vi "Fetch (PV Data).vi"(7 "PV name":string, 8 "error in":errorcluster, 11 "Source in":refnum<class "Source.lvclass">) -> (0 "error out":errorcluster, 1 "PV found?":bool, 2 "PV Data out":refnum<class "PV Data.lvclass">, 3 "Source out":refnum<class "Source.lvclass">)   [LabVIEW 2020, in "PV Access.lvlib" / "PVA Server.lvlib" / "Source.lvclass"]
uses:
  Source.lvclass
  PV Data/PV Data/PV Data.lvclass
  Source.lvclass/Source.ctl
  PV Access.lvlib
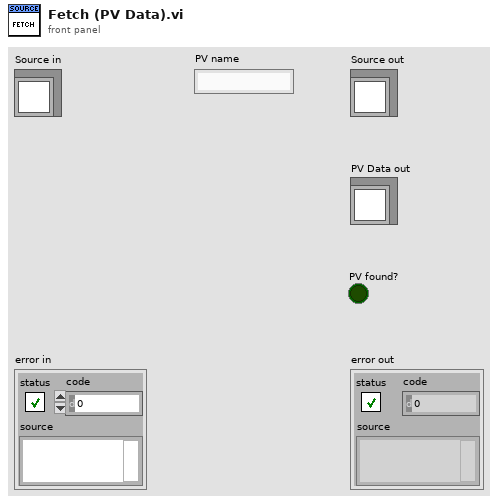
[diagram p1: front panel]
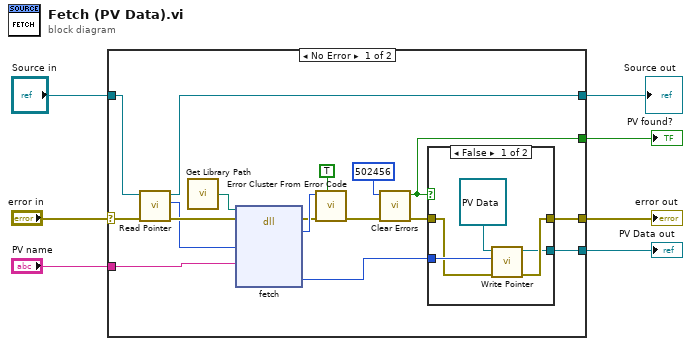
[diagram p0: block diagram]
diagram:
  n1 = case shown="No Error" "error in" {
    selector: "error in" -> [w24 w32]
    tunnel: [w14 w32] -> w6
    tunnel: [w20 w31] -> w2
    tunnel: "PV name" -> [w19 _]
    tunnel: [w13 _] -> w4
    tunnel: "Source in" -> [w15 w31]
    tunnel: [w8 _] -> w1
    frame No Error {
      n2 = call-dynamic "Read Pointer.vi"("error in (no error)"=w24, "Pointer Base in"=w15) -> ("error out"=w23:errorcluster, "Pointer"=w21:i64, "Pointer Base out"=w20:refnum<class "Source.lvclass">)  [unwired: 7 in]
      n3 = call "Get Library Path.vi"() -> ("Path"=w22:path)  [unwired: 1 in]
      n4 = dll-call lib="?" fn="fetch"(path in=w22, error in=w23, "source"=w21, "pv_name"=w19) -> (error out=w16:errorcluster, "ret_code"=w17:i32, "value"=w12:i64)  [unwired: 4 in, 1 out]
      n5 = call <vilib>:"Error Cluster From Error Code.vi"("show call chain? (False)"=TRUE, "error in (no error)"=w16, "error code (0)"=w17) -> ("error out"=w11:errorcluster)  [unwired: 6 in]
      n6 = call <vilib>:"Clear Errors.vi"("error in (no error)"=w11, "specific error code to clear (0: all)"=502456) -> ("error out"=w10:errorcluster, "specific error cleared?"=w8:bool)  [unwired: 4 in]
      n7 = case shown="False" w8 {
        tunnel: [w29 w30] -> w14
        tunnel: [w28 _] -> w13
        tunnel: w12 -> [w26 _]
        tunnel: w10 -> [w25 w30]
        frame False {
          n8 = call-dynamic "Write Pointer.vi"("error in (no error)"=w25, "Pointer"=w26, "Pointer Base in"=refnum<class "PV Data.lvclass"> refnum ("PV Access.lvlib:PV Data.lvlib:PV Data.lvclass")) -> ("error out"=w29:errorcluster, "Pointer Base out"=w28:refnum<class "PV Data.lvclass">)  [unwired: 7 in]
        }
        frame True {
        }
      }
    }
    frame Error {
    }
  }
  "error out" <- w6
  "PV Data out" <- w4
  "Source out" <- w2
  "PV found?" <- w1
